vi "updateTemperature.vi"(8 "error in (no error)":errorcluster, 11 "AndorIKonTempController in":refnum<class "AndorIKonTempController.lvclass">) -> (0 "error out":errorcluster, 1 "Status":string, 2 "updateTemperature":dbl, 3 "AndorIKonTempController out":refnum<class "AndorIKonTempController.lvclass">)   [LabVIEW 2011, in "Hardware.lvlib" / "Channels.lvlib" / "AndorIKonTempController.lvclass"]
doc: "Gets the current temperature of the Andor camera, and returns the status of the cooling. If the camera has reached the set point, has not reaached the set point, has drifted from it, etc."
uses:
  AndorIKonTempController.lvclass
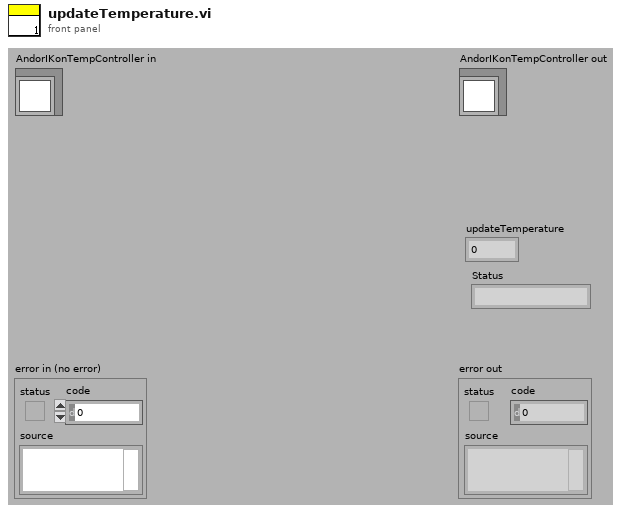
[diagram p1: front panel]
types:
  T1 = typedef "Error Code Enum typedef.ctl" = enum32{"N/A (0)", "DRV_ERROR_CODES", "DRV_SUCCESS", "DRV_VXDNOTINSTALLED", "DRV_ERROR_SCAN", "DRV_ERROR_CHECK_SUM", "DRV_ERROR_FILELOAD", "DRV_UNKNOWN_FUNC", "DRV_ERROR_VXD_INIT", "DRV_ERROR_ADDRESS", "DRV_ERROR_PAGELOCK", "DRV_ERROR_PAGEUNLOCK", "DRV_ERROR_BOARDTEST", "DRV_ERROR_ACK", "DRV_ERROR_UP_FIFO", "DRV_ERROR_PATTERN", "N/A (16)", "DRV_ACQUISITION_ERRORS", "DRV_ACQ_BUFFER", "DRV_ACQ_DOWNFIFO_FULL", "DRV_PROC_UNKONWN_INSTRUCTION", "DRV_ILLEGAL_OP_CODE", "DRV_KINETIC_TIME_NOT_MET", "DRV_ACCUM_TIME_NOT_MET", "DRV_NO_NEW_DATA", "N/A (25)", "DRV_SPOOLERROR", "N/A (27)", "N/A (28)", "N/A (29)", "N/A (30)", "N/A (31)", "N/A (32)", "DRV_TEMPERATURE_CODES", "DRV_TEMPERATURE_OFF", "DRV_TEMPERATURE_NOT_STABILIZED", "DRV_TEMPERATURE_STABILIZED", "DRV_TEMPERATURE_NOT_REACHED", "DRV_TEMPERATURE_OUT_RANGE", "DRV_TEMPERATURE_NOT_SUPPORTED", "DRV_TEMPERATURE_DRIFT", "N/A (41)", "N/A (42)", "N/A (43)", "N/A (44)", "N/A (45)", "N/A (46)", "N/A (47)", "N/A (48)", "DRV_GENERAL_ERRORS", "DRV_INVALID_AUX", "DRV_COF_NOTLOADED", "DRV_FPGAPROG", "DRV_FLEXERROR", "DRV_GPIBERROR", "N/A (55)", "N/A (56)", "N/A (57)", "N/A (58)", "N/A (59)", "N/A (60)", "N/A (61)", "N/A (62)", "N/A (63)", "DRV_DATATYPE", "DRV_DRIVER_ERRORS", "DRV_P1INVALID", "DRV_P2INVALID", "DRV_P3INVALID", "DRV_P4INVALID", "DRV_INIERROR", "DRV_COFERROR", "DRV_ACQUIRING", "DRV_IDLE", "DRV_TEMPCYCLE", "DRV_NOT_INITIALIZED", "DRV_P5INVALID", "DRV_P6INVALID", "DRV_INVALID_MODE", "DRV_INVALID_FILTER", "DRV_I2CERRORS", "DRV_I2CDEVNOTFOUND", "DRV_I2CTIMEOUT", "DRV_P7INVALID", "N/A (84)", "N/A (85)", "N/A (86)", "N/A (87)", "N/A (88)", "N/A (89)", "DRV_IOCERROR", "DRV_VRMVERSIONERROR"}
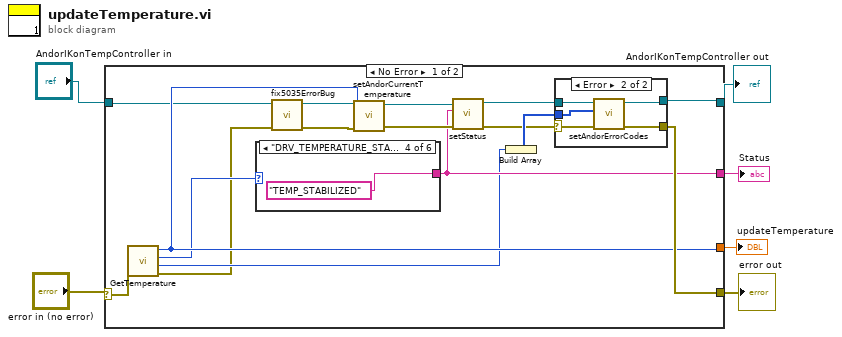
[diagram p0: block diagram]
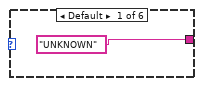
[diagram p2: hidden frame]
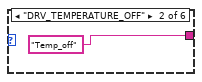
[diagram p3: hidden frame]
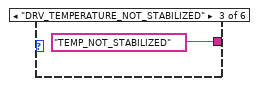
[diagram p4: hidden frame]
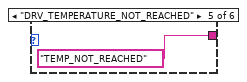
[diagram p5: hidden frame]
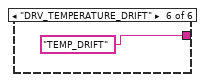
[diagram p6: hidden frame]
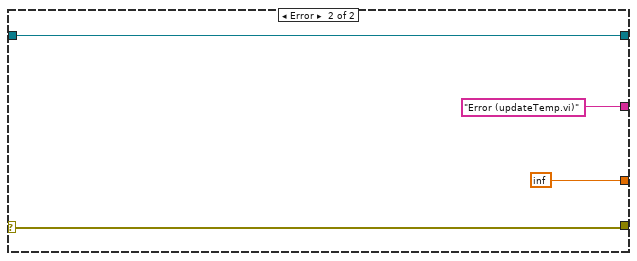
[diagram p8: hidden frame]
diagram:
  n1 = case shown="No Error" "error in (no error)" {
    selector: "error in (no error)" -> [w22 w39]
    tunnel: [w20 w39] -> w5
    tunnel: "AndorIKonTempController in" -> [w7 w38]
    tunnel: [w21 w38] -> w3
    tunnel: [w18 inf] -> w2
    tunnel: [w12 "Error (updateTemp.vi)"] -> w1
    frame No Error {
      n2 = call <userlib>:"GetTemperature.vi"("error in (no error)"=w22) -> ("error out"=w8:errorcluster, "DLL error code"=w11:u32, "status"=w13:T1, "temperature"=w18:i32)  [unwired: 3 in]
      n3 = case shown="\"DRV_TEMPERATURE_STABILIZED\"" w13 {
        tunnel: ["UNKNOWN" "Temp_off" "TEMP_NOT_STABILIZED" "TEMP_STABILIZED" "TEMP_NOT_REACHED" "TEMP_DRIFT"] -> w12
        frame Default {
        }
        frame "DRV_TEMPERATURE_OFF" {
        }
        frame "DRV_TEMPERATURE_NOT_STABILIZED" {
        }
        frame "DRV_TEMPERATURE_STABILIZED" {
        }
        frame "DRV_TEMPERATURE_NOT_REACHED" {
        }
        frame "DRV_TEMPERATURE_DRIFT" {
        }
      }
      n4 = call "fix5035ErrorBug.vi"("error in (no error)"=w8, "AndorIKonTempController in"=w7) -> ("error out"=w9:errorcluster, "AndorIKonTempController out"=w10:refnum<class "AndorIKonTempController.lvclass">)  [unwired: 8 in]
      n5 = call "setAndorCurrentTemperature.vi"("error in (no error)"=w9, "currentTemperature"=w18, "AndorIKonTempController.lvclass in"=w10) -> ("error out"=w17:errorcluster, "AndorIKonTempController.lvclass out"=w16:refnum<class "AndorIKonTempController.lvclass">)  [unwired: 7 in]
      n6 = call "setStatus.vi"("error in (no error)"=w17, "Status"=w12, "AndorIKonTempController.lvclass in"=w16) -> ("error out"=w14:errorcluster, "AndorIKonTempController.lvclass out"=w15:refnum<class "AndorIKonTempController.lvclass">)  [unwired: 7 in]
      n7 = Build Array(w11) -> (w19:u32[])
      n8 = case shown="Error" w14 {
        selector: w14 -> [w30 w33]
        tunnel: w15 -> [w29 w35]
        tunnel: [w29 w34] -> w21
        tunnel: [w30 w32] -> w20
        tunnel: w19 -> [_ w31]
        frame No Error {
        }
        frame Error {
          n9 = call-dynamic "setAndorErrorCodes.vi"("error in (no error)"=w33, "Andor Error Codes"=w31, "AndorIKonTempController.lvclass in"=w35) -> ("error out"=w32:errorcluster, "AndorIKonTempController.lvclass out"=w34:refnum<class "AndorIKonTempController.lvclass">)  [unwired: 7 in]
        }
      }
    }
    frame Error {
    }
  }
  "error out" <- w5
  "AndorIKonTempController out" <- w3
  "updateTemperature" <- w2
  "Status" <- w1
